vi "Control Styles.vi"() -> ()   [LabVIEW 2020]
panel:
  out "String 10":string
  in  "String 9":string
  out "Boolean 8":bool
  in  "Boolean 7":bool
  out "Numeric 10":dbl
  in  "Numeric 9":dbl
  out "String 8":string
  in  "String 7":string
  in  "Boolean 6":bool
  in  "Numeric 8":dbl
  in  "Numeric 7":dbl
  out "String 6":string
  in  "String 5":string
  out "Boolean 5":bool
  in  "Boolean 4":bool
  out "Numeric 6":dbl
  in  "Numeric 5":dbl
  out "String 4":string
  in  "String 3":string
  out "Boolean 3":bool
  in  "Button":bool
  out "Numeric 4":dbl
  in  "Numeric 3":dbl
  out "String 2":string
  in  "String":string
  out "Boolean 2":bool
  in  "Boolean":bool
  out "Numeric 2":dbl
  in  "Numeric":dbl
  # "Modern"
  # "NXG Style"
  # "Sliver"
  # "System"
  # "Classic"
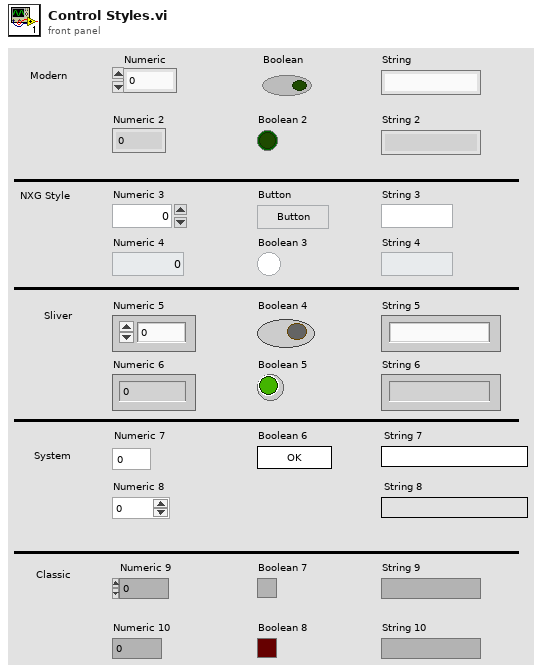
[diagram p1: front panel]
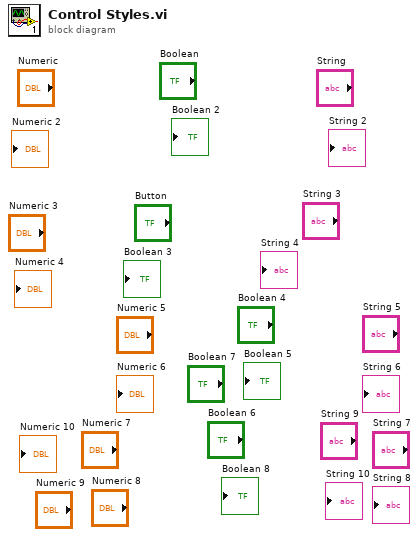
[diagram p0: block diagram]
diagram:
